vi "CheckDBConnection.vi"(3 "error in (no error)":errorcluster, 5 "LotData in":refnum<class "LotData.lvclass">) -> (0 "error out":errorcluster, 1 "ConnectionError?":bool, 2 "LotData out":refnum<class "LotData.lvclass">)   [LabVIEW 2012, in "LotData.lvclass"]
uses:
  LotData.lvclass
  LotData.lvclass/LotData.ctl
  <vilib>/addons/database/Connection.llb/DB Tools Open Connec (Path).vi
  <vilib>/addons/database/NI_Database_API.lvlib
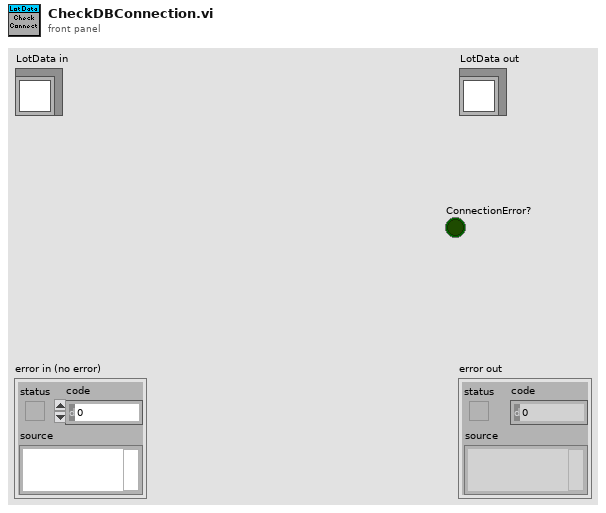
[diagram p1: front panel]
types:
  T1 = typedef "NI_Database_API.lvlib/Conn ObjectReference.ctl" = refnum<k1>
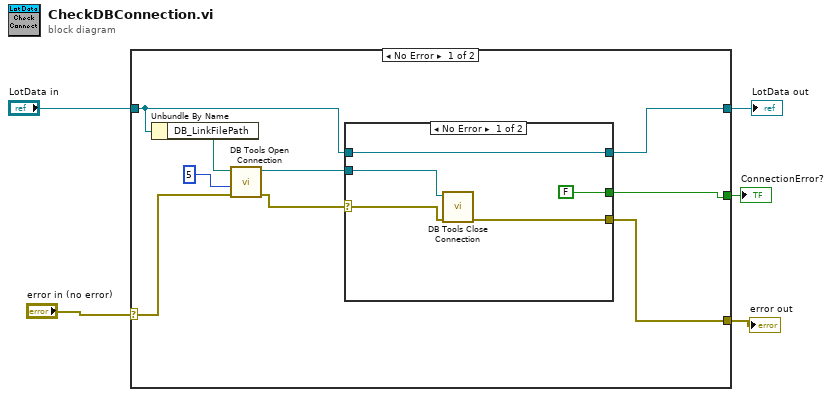
[diagram p0: block diagram]
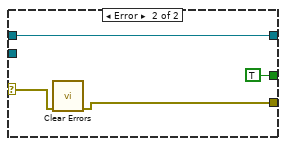
[diagram p2: hidden frame]
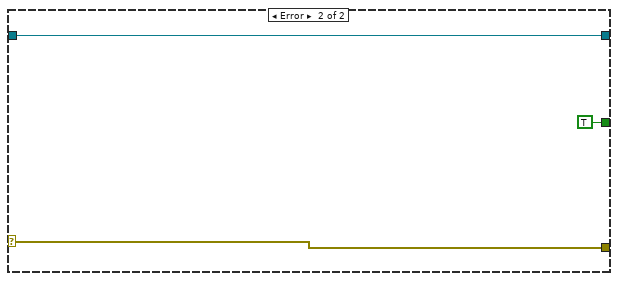
[diagram p3: hidden frame]
diagram:
  n1 = case shown="No Error" "error in (no error)" {
    selector: "error in (no error)" -> [w13 w26]
    tunnel: [w9 w26] -> w4
    tunnel: [w8 w25] -> w2
    tunnel: "LotData in" -> [w7 w25]
    tunnel: [w6 TRUE] -> w1
    frame No Error {
      n2 = Unbundle By Name(w7) -> ("DB_LinkFilePath"=w14:path)
      n3 = call-poly <vilib>:"DB Tools Open Connection.vi"("error in (no error)"=w13, "connection timeout (15)"=5, "connection information"=w14) -> ("error out"=w11:errorcluster, "connection reference"=w10:T1)  [unwired: 5 in]
      n4 = case shown="No Error" w11 {
        selector: w11 -> [w18 w22]
        tunnel: w10 -> [w19 _]
        tunnel: [w17 w21] -> w9
        tunnel: [w16 w23] -> w8
        tunnel: w7 -> [w16 w23]
        tunnel: [FALSE TRUE] -> w6
        frame No Error {
          n5 = call <vilib>:"DB Tools Close Connection.vi"("error in (no error)"=w18, "connection reference"=w19) -> ("error out"=w17:errorcluster)  [unwired: 5 in]
        }
        frame Error {
          n6 = call <vilib>:"Clear Errors.vi"("error in (no error)"=w22) -> ("error out"=w21:errorcluster)  [unwired: 6 in]
        }
      }
    }
    frame Error {
    }
  }
  "error out" <- w4
  "LotData out" <- w2
  "ConnectionError?" <- w1
